vi "Write MAG.vi"(8 "error in (no error)":errorcluster, 10 "MAG":dbl, 11 "Referential in":refnum<class "Referential.lvclass">) -> (0 "error out":errorcluster, 3 "Referential out":refnum<class "Referential.lvclass">)   [LabVIEW 2019, in "Referential.lvclass"]
uses:
  Referential.lvclass
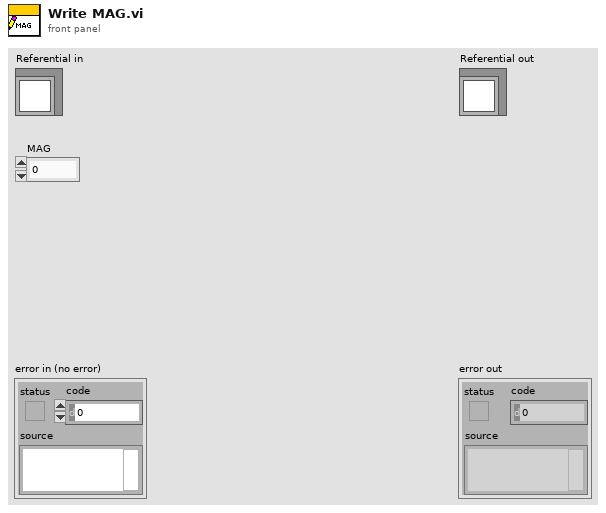
[diagram p1: front panel]
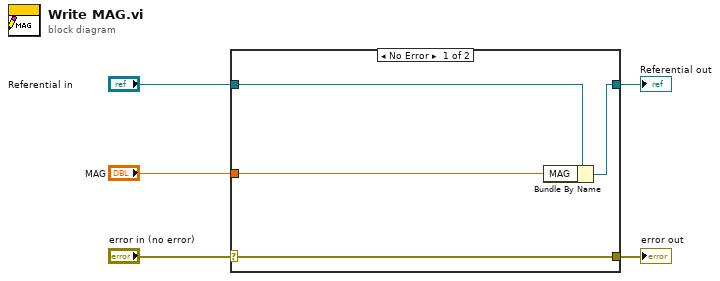
[diagram p0: block diagram]
diagram:
  n1 = case shown="No Error" "error in (no error)" {
    selector: "error in (no error)" -> [w9 w10]
    tunnel: [w9 w10] -> w4
    tunnel: [w7 w11] -> w2
    tunnel: "Referential in" -> [w8 w11]
    tunnel: "MAG" -> [w6 _]
    frame No Error {
      n2 = Bundle By Name(cluster=w8, "MAG"=w6) -> (w7:refnum<class "Referential.lvclass">)
    }
    frame Error {
    }
  }
  "error out" <- w4
  "Referential out" <- w2
